vi "Cure Target.vi"() -> ()   [LabVIEW 2017, in "Tests.lvlib"]
uses:
  Tests.lvlib
panel:
  in  "Input":bool[](array[boolean])=[FALSE, FALSE, FALSE, TRUE, FALSE, FALSE]
  out "Any?":bool
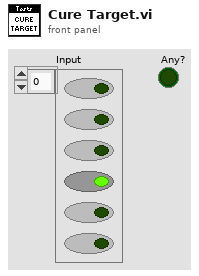
[diagram p1: front panel]
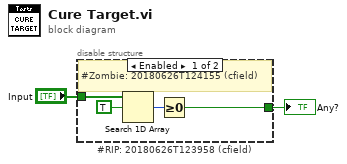
[diagram p0: block diagram]
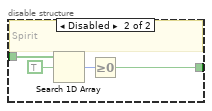
[diagram p2: hidden frame]
diagram:
  n1 = disable-structure "#RIP: 20180626T123958 (cfield)" shown="Enabled" {
    disable-tunnel: "Input" -> [w6 w10]
    disable-tunnel: [w5 w9] -> w1
    frame Enabled {
      # "#Zombie: 20180626T124155 (cfield)"
      n2 = Search 1D Array(1D array=w6, element=TRUE) -> (index of element=w3:i32)  [unwired: 1 in]
      n3 = Greater Or Equal To 0?(x=w3) -> (x >= 0?=w5:bool)
    }
    frame Disabled {
      # "Spirit"
      n4 = Search 1D Array(1D array=w10, element=TRUE) -> (index of element=w7:i32)  [unwired: 1 in]
      n5 = Greater Or Equal To 0?(x=w7) -> (x >= 0?=w9:bool)
    }
  }
  "Any?" <- w1
